vi "AirHockey.vi"() -> ()   [LabVIEW 2017]
panel:
  out "new picture":picture caption="Air Hockey"
  in  "C2":u32(colorbox)=65302
  in  "pause":i32=10
  in  "C3":u32(colorbox)=16395007
  out "error out 2":errorcluster
  in  "Seq":string
  out "sortie d'erreur":errorcluster
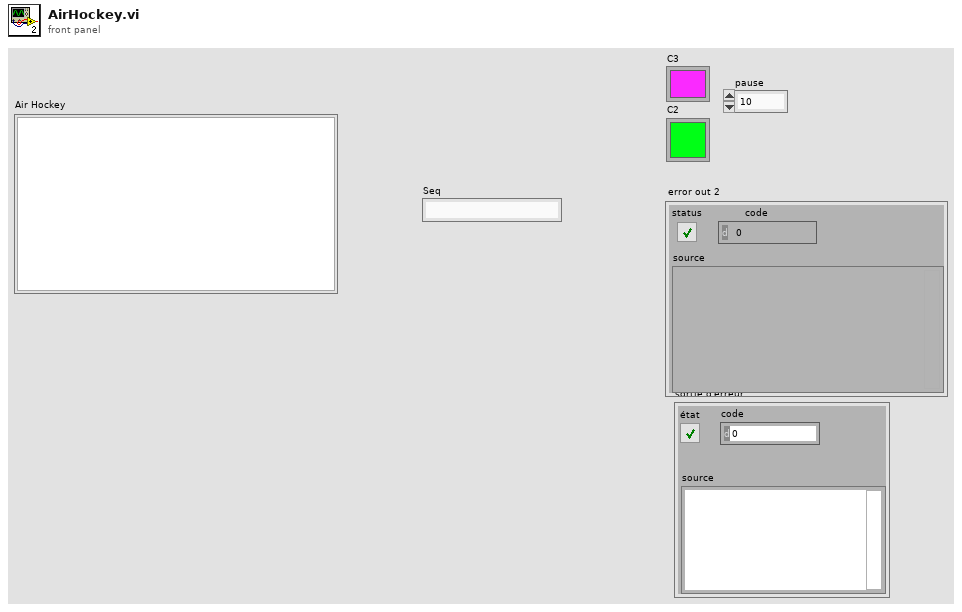
[diagram p1: front panel]
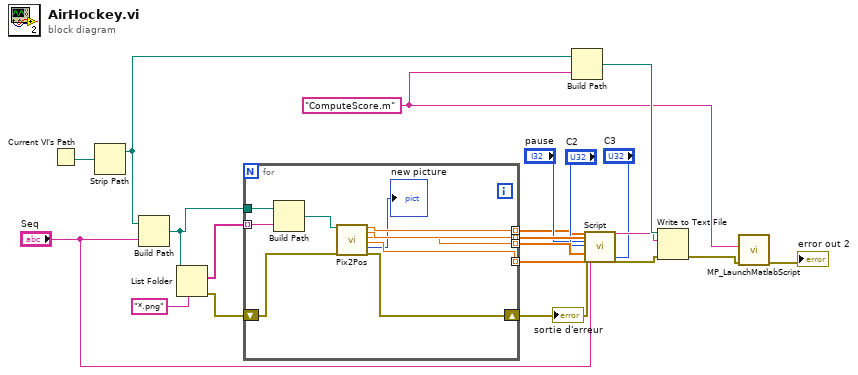
[diagram p0: block diagram]
diagram:
  w11 = "ComputeScore.m" ("ComputeScore.m")
  n1 = Current VI's Path() -> (path=w5:path)
  n2 = Strip Path(path=w5) -> (stripped path=w17:path)  [unwired: 1 out]
  n3 = Build Path(base path=w17, name or relative path="Seq") -> (appended path=w19:path)
  n4 = List Folder(path=w19, pattern="*.png" ("filtre")) -> (filenames=w20:string[], error out=w18:errorcluster)  [unwired: 2 in, 2 out]
  n5 = for {
    tunnel: w20 -> [w31] mode=indexing
    tunnel: w19 -> [w30]
    tunnel: [w25] -> w8 mode=indexing
    tunnel: [w24] -> w7 mode=indexing
    shift-right: [w28] -> w15
    shift-left: w18 -> [w29]
    tunnel: [w26] -> w1 mode=indexing
    tunnel: [w23] -> w6 mode=indexing
    n6 = Build Path(base path=w30, name or relative path=w31) -> (appended path=w27:path)
    n7 = call "Pix2Pos.vi"("Chemin vers le fichier PNG"=w27, "entrée d'erreur"=w29) -> ("X1"=w26:dbl, "Y1"=w25:dbl, "X2"=w24:dbl, "Y2"=w23:dbl, "new picture"=→"new picture":picture, "sortie d'erreur"=w28:errorcluster)  [unwired: 12 in]
  }
  "sortie d'erreur" <- w15
  n8 = Build Path(base path=w17, name or relative path=w11) -> (appended path=w16:path)
  n9 = call "Script.vi"("entrée 1"=w1, "entrée 2"=w8, "pause"="pause", "C2"="C2", "entrée d'erreur"=w15, "entrée 3"=w7, "C3"="C3", "entrée 4"=w6, "Seq"="Seq") -> ("SCRIPT FINAL"=w12:string, "sortie d'erreur"=w13:errorcluster)  [unwired: 17 in]
  n10 = Write to Text File(file (use dialog)=w16, text=w12, error in=w13) -> (error out=w9:errorcluster)  [unwired: 1 in, 2 out]
  n11 = call "MP_LaunchMatlabScript.vi"("error in (no error)"=w9, "matlab script name with extension"=w11) -> ("error out"=→"error out 2":errorcluster)  [unwired: 5 in, 4 out]
